vi "proc.util.enumToStrIoConfvi.vi"(10 "Step var":T1) -> (2 "String":string)   [LabVIEW 2024]
uses:
  controls/enum.io-rio.ctl
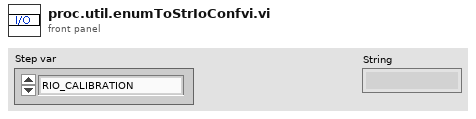
[diagram p1: front panel]
types:
  T1 = typedef "enum.io-rio.ctl" = enum16{"RIO_CALIBRATION"}
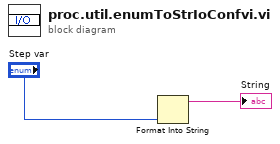
[diagram p0: block diagram]
diagram:
  n1 = Format Into String("Step var") -> (resulting string=→"String":string)  [unwired: 3 in, 1 out]
